vi "MessageName.vi"() -> (2 "MessageName":string)   [LabVIEW 2020, in "StartSeq.lvlib"]
uses:
  StartSeq.lvlib
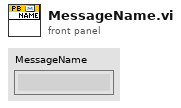
[diagram p1: front panel]
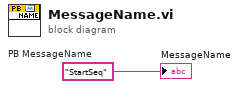
[diagram p0: block diagram]
diagram:
  w1 = "StartSeq"  # PB MessageName
  "MessageName" <- w1
